vi "Start.vi"(8 "error in":errorcluster, 11 "AO DAQmx DC CFG in":refnum<class "AO DAQmx DC CFG.lvclass">) -> (0 "error out":errorcluster, 3 "AO DAQmx DC CFG out":refnum<class "AO DAQmx DC CFG.lvclass">)   [LabVIEW 2023, in "AO DAQmx DC CFG.lvclass"]
uses:
  AO DAQmx DC CFG.lvclass
  Configuration/Configuration JSON/Configuration JSON Base/CFG JSON.lvclass/CFG JSON.ctl
  DAQmx/DAQmx Base CFG/DAQmx Base CFG.lvclass/DAQmx Base CFG.ctl
  AO DAQmx DC CFG.lvclass/AO DAQmx DC CFG.ctl
  <vilib>/DAQmx/miscellaneous.llb/DAQmx Fill In Error Info.vi
  <vilib>/DAQmx/write.llb/DAQmx Write (Analog 1D DBL NChan 1Samp).vi
  DAQmx/BufferWrites1SamDBL/BufferWrites1SamDBL.lvclass
  DAQmx/DAQmx Base CFG/DAQmx Base CFG.lvclass
  Configuration/Configuration JSON/Configuration JSON Base/CFG JSON.lvclass
  D:/git/HAL/HAL GOOP4/DAQmx/DAQmx Base CFG/DAQmx Base CFG.lvclass
  D:/git/HAL/HAL GOOP4/CFG Target/CFG Target.lvclass
  D:/git/HAL/HAL GOOP4/Configuration/Configuration Semaphore/CFG Semaphore.lvclass
  D:/git/HAL/HAL GOOP4/Configuration/Configuration JSON/Configuration JSON Base/CFG JSON.lvclass
  D:/git/HAL/HAL GOOP4/Interfaces/IConfigure/IConfigure.lvclass
  D:/git/HAL/HAL GOOP4/AO/AO DAQmx DC CFG/AO DAQmx DC CFG.lvclass
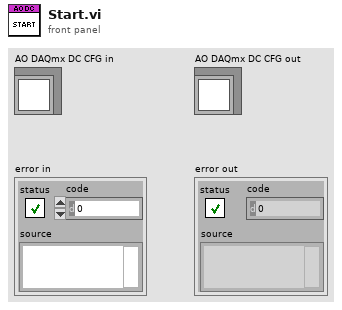
[diagram p1: front panel]
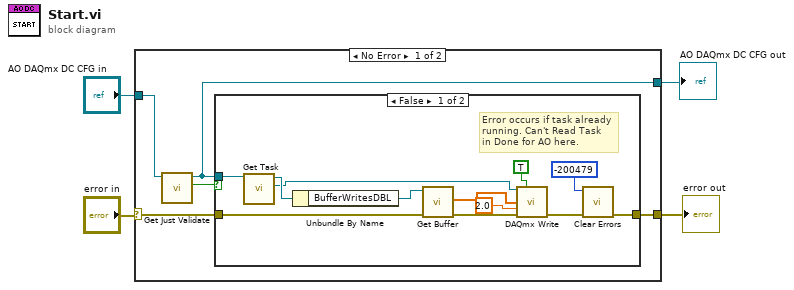
[diagram p0: block diagram]
diagram:
  n1 = case shown="No Error" "error in" {
    selector: "error in" -> [w7 w24]
    tunnel: "AO DAQmx DC CFG in" -> [w8 w23]
    tunnel: [w6 w23] -> w1
    tunnel: [w9 w24] -> w2
    frame No Error {
      n2 = call "Get Just Validate.vi"("CFG JSON Base in"=w8) -> ("Just Validate"=w5:bool, "CFG JSON Base out"=w6:refnum<class "AO DAQmx DC CFG.lvclass">)  [unwired: 9 in]
      n3 = case shown="False" w5 {
        tunnel: [w11 w22] -> w9
        tunnel: w7 -> [w20 w22]
        tunnel: w6 -> [w19 _]
        frame False {
          # "Error occurs if task already\nrunning. Can't Read Task\nin Done for AO here."
          n4 = call "Get Task.vi"("DAQmx Base CFG in"=w19) -> ("Task"=w17:refnum<k21>, "DAQmx Base CFG out"=w18:refnum<class "AO DAQmx DC CFG.lvclass">)  [unwired: 9 in]
          n5 = Unbundle By Name(w18) -> ("BufferWritesDBL"=w16:refnum<class "BufferWrites1SamDBL.lvclass">)
          n6 = call "Get Buffer.vi"("error in"=w20, "BufferWrites1SamDBL in"=w16) -> ("error out"=w14:errorcluster, "Buffer"=w13:dbl[])  [unwired: 7 in, 1 out]
          n7 = call-poly <vilib>:"DAQmx Write.vi"("task/channels in"=w17, "auto start"=TRUE, "data"=w13, "timeout"=2.0, "error in"=w14) -> ("error out"=w21:errorcluster)  [unwired: 8 in, 2 out]
          n8 = call <vilib>:"Clear Errors.vi"("error in (no error)"=w21, "specific error code to clear (0: all)"=-200479) -> ("error out"=w11:errorcluster)  [unwired: 4 in, 1 out]
        }
        frame True {
        }
      }
    }
    frame Error {
    }
  }
  "error out" <- w2
  "AO DAQmx DC CFG out" <- w1
